vi "ADIS16470 Loop.vi"(8 "error in":errorcluster) -> ()   [LabVIEW 2018]
uses:
  Typedef/ADIS16470 Device Reference.ctl
  Typedef/ADIS16470 Hardware Configuration.ctl
  <vilib>/Rock Robotics/WPI/SPI/WPI_SPIMode.ctl
  <vilib>/Rock Robotics/SystemInterfaces/DIO/FPGA_DIOChannel.ctl
  <vilib>/Rock Robotics/SystemInterfaces/spilib/spi_bus.ctl
  Typedef/ADIS16470 Data.ctl
  Typedef/ADIS16470 Status.ctl
  Typedef/ADIS16470 Process.ctl
  Typedef/ADIS16470 Command Type.ctl
  <vilib>/Rock Robotics/WPI/SPI/WPI_SPIDevRef.ctl
  <vilib>/Rock Robotics/WPI/Interrupt/WPI_InterruptRef.ctl
  <vilib>/Rock Robotics/SystemInterfaces/Interrupt/FPGA_InterruptIndex.ctl
  Typedef/ADIS16470 Register.ctl
  <vilib>/Rock Robotics/WPI/Counter/WPI_CounterDigitalInputToDigitalSource.vi
  <vilib>/Rock Robotics/SystemInterfaces/CounterEncoderSourceConvertion/FPGA_CounterEncoderSourceConvertionLVSourceTypeToFPGAType.vi
  <vilib>/Rock Robotics/WPI/Interrupt/WPI_InterruptCache.vi
  <vilib>/Rock Robotics/SystemInterfaces/Interrupt/FPGA_InterruptWriteConfiguration.vi
  <vilib>/Rock Robotics/SystemInterfaces/Interrupt/FPGA_WaitOnInterrupt.vi
  <vilib>/Rock Robotics/WPI/Utilities/WPI_UtilitiesTimebaseConstants.vi
  <vilib>/Rock Robotics/SystemInterfaces/Interrupt/FPGA_InterruptReadTimestamp.vi
panel:
  out "Waveform Chart":dbl(graph)
  out "Offset Bias":i16[](array[numeric])
  out "xAngle":dbl
  out "yAngle":dbl
  out "Data":dbl[](array[numeric])
  out "Counter":u16
  in  "ADIS16470DevRef":T1={"DevStatus"={"status"=FALSE, "code"=0, "source"=""}, "Hardware Config"={"SPI Clock Rate (Hz)"=1000000.0, "IMU SPI Mode (3)"=enum."Mode 3 (Clk Idle High,Sample on Trailing)", "IMU Reset Pin"=enum."SPI Port CS2", "IMU SPI Bus"=enum."SPI On-Board, CS0", "IMU Data Ready Pin"=enum."SPI Port CS1"}, "End Calibration"=refnum, "Calibration Complete"=refnum, "Data FIFO"=refnum, "Status FIFO"=refnum, "Last Value Reference"=refnum, "Sychronous Process VI"=refnum, "Cmd FIFO"=refnum}
  in  "Main Name":string
  # "x"
  # "y"
  # "z"
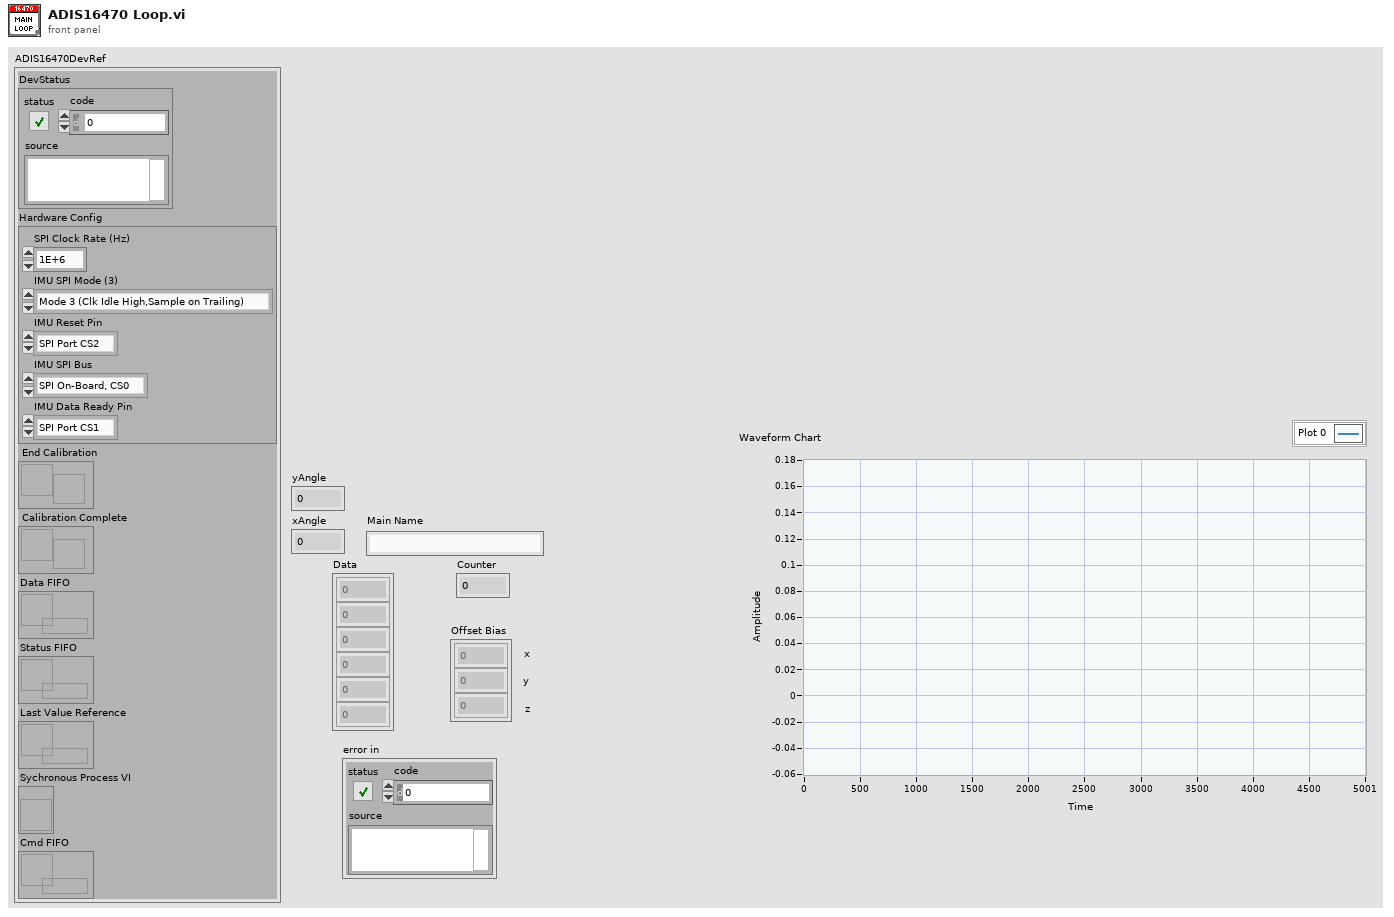
[diagram p1: front panel]
types:
  T1 = typedef "ADIS16470 Device Reference.ctl" = cluster{"DevStatus":errorcluster, "Hardware Config":T2, "End Calibration":refnum<notifier>, "Calibration Complete":refnum<notifier>, "Data FIFO":refnum<k33>, "Status FIFO":refnum<k33>, "Last Value Reference":refnum<data-value>, "Sychronous Process VI":T6, "Cmd FIFO":refnum<k33>}
  T2 = typedef "ADIS16470 Hardware Configuration.ctl" = cluster{"SPI Clock Rate (Hz)":dbl, "IMU SPI Mode (3)":T3, "IMU Reset Pin":T4, "IMU SPI Bus":T5, "IMU Data Ready Pin":T4}
  T3 = typedef "WPI_SPIMode.ctl" = enum16{"Mode 0 (Clk Idle Low,Sample on Leading)", "Mode 1 (Clk Idle Low,Sample on Trailing)", "Mode 2 (Clk Idle High,Sample on Leading)", "Mode 3 (Clk Idle High,Sample on Trailing)"}
  T4 = typedef "FPGA_DIOChannel.ctl" = enum8{"DIO 0", "DIO 1", "DIO 2", "DIO 3", "DIO 4", "DIO 5", "DIO 6", "DIO 7", "DIO 8", "DIO 9", "DIO MXP 0", "DIO MXP 1", "DIO MXP 2", "DIO MXP 3", "DIO MXP 4", "DIO MXP 5", "DIO MXP 6", "DIO MXP 7", "DIO MXP 8", "DIO MXP 9", "DIO MXP 10", "DIO MXP 11", "DIO MXP 12", "DIO MXP 13", "DIO MXP 14", "DIO MXP 15", "SPI Port CS1", "SPI Port CS2", "SPI Port CS3", "SPI Port MISO", "SPI Port MOSI", "Invalid"}
  T5 = typedef "spi_bus.ctl" = enum16{"SPI On-Board, CS0", "SPI On-Board, CS1", "SPI On-Board, CS2", "SPI On-Board, CS3", "SPI MXP", "Invalid"}
  T6 = typedef "ADIS16470 Process.ctl" = refnum<vi>
  T7 = typedef "WPI_SPIDevRef.ctl" = cluster{"DevStatus":errorcluster, "Handle":i32, "SPI Bus":T5}
  T8 = typedef "WPI_InterruptRef.ctl" = cluster{"DevStatus":errorcluster, "InterruptIndex":T9}
  T9 = typedef "FPGA_InterruptIndex.ctl" = enum8{"0", "1", "2", "3", "4", "5", "6", "7", "Invalid"}
  T10 = cluster{"ADIS16470DevRef":T1, "SPIDevRef":T7, "InterruptRef":T8, "Sensor to Robot Rotation":dbl[][], "Yaw":dbl, "Data Counter":u16, "First Run":bool, "TimeStamp Prev":dbl, "Time Delta":dbl}
  T11 = typedef "ADIS16470 Status.ctl" = cluster{"Calibrated?":bool}
  T12 = typedef "ADIS16470 Register.ctl" = u8
  T13 = typedef "ADIS16470 Command Type.ctl" = enum16{"None", "Reset"}
  T14 = typedef "ADIS16470 Data.ctl" = cluster{"Yaw":dbl, "Timestamp":dbl, "Timestamp Delta":dbl, "Sample Count":u16}
  T15 = typedef "WPI_DigitalOutputDevRef.ctl" = cluster{"DIO Channel":T4, "DevStatus":errorcluster}
  T16 = typedef "WPI_DigitalInputDevRef.ctl" = cluster{"DevStatus":errorcluster, "DIO Channel":T4}
  T17 = typedef "FPGA_CounterEncoderSourceConvertionLVSourceType.ctl" = cluster{"DevStatus":errorcluster, "AnalogTriggerMode?":bool, "DigitalMode":cluster{"DIO Channel":T18}, "AnalogTriggerMode":cluster{"AnalogTriggerIndex":T19, "OutputType":T20}}
  T18 = typedef "FPGA_DIODigitalSourceChannel.ctl" = enum8{"DIO 0", "DIO 1", "DIO 2", "DIO 3", "DIO 4", "DIO 5", "DIO 6", "DIO 7", "DIO 8", "DIO 9", "DIO MXP 0", "DIO MXP 1", "DIO MXP 2", "DIO MXP 3", "DIO MXP 4", "DIO MXP 5", "DIO MXP 6", "DIO MXP 7", "DIO MXP 8", "DIO MXP 9", "DIO MXP 10", "DIO MXP 11", "DIO MXP 12", "DIO MXP 13", "DIO MXP 14", "DIO MXP 15", "SPI Port CS1", "SPI Port CS2", "SPI Port CS3", "SPI Port MISO", "SPI Port MOSI", "Disabled"}
  T19 = typedef "FPGA_AnalogTriggerIndex.ctl" = enum8{"Trig 0", "Trig 1", "Trig 2", "Trig 3", "Trig 4", "Trig 5", "Trig 6", "Trig 7", "Invalid"}
  T20 = typedef "FPGA_AnalogTriggerOutType.ctl" = enum16{"InWindow", "TriggerState", "Rising", "Falling"}
  T21 = enum32{"Bad", "Idle", "Run top level", "Running"}
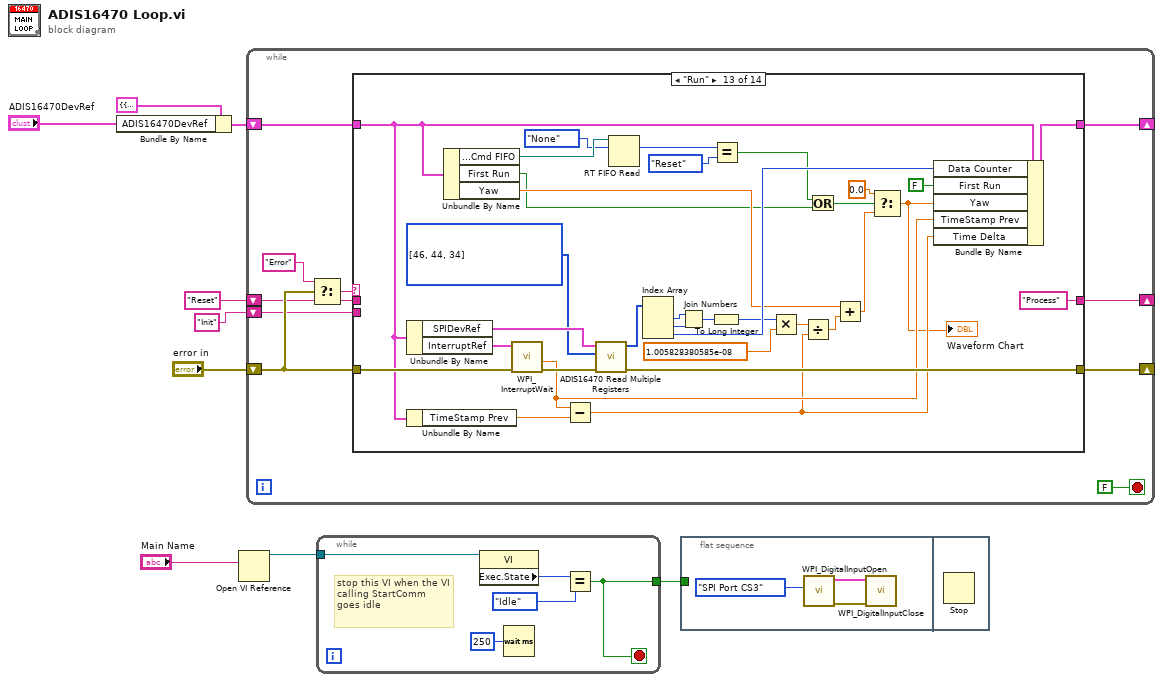
[diagram p0: block diagram]
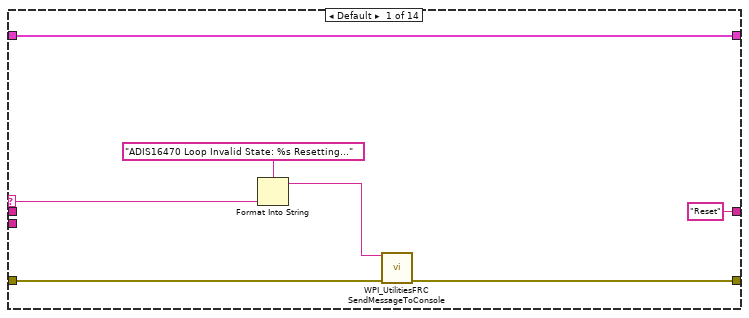
[diagram p2: hidden frame]
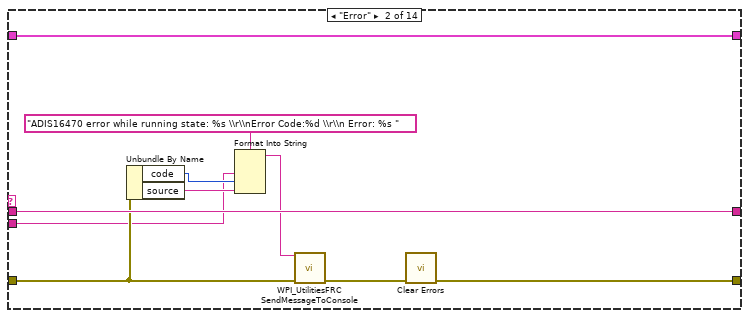
[diagram p3: hidden frame]
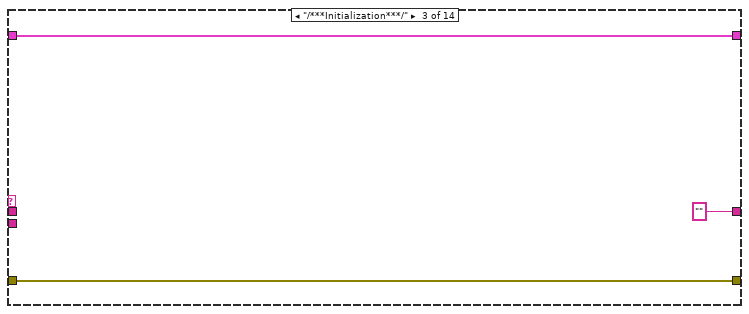
[diagram p4: hidden frame]
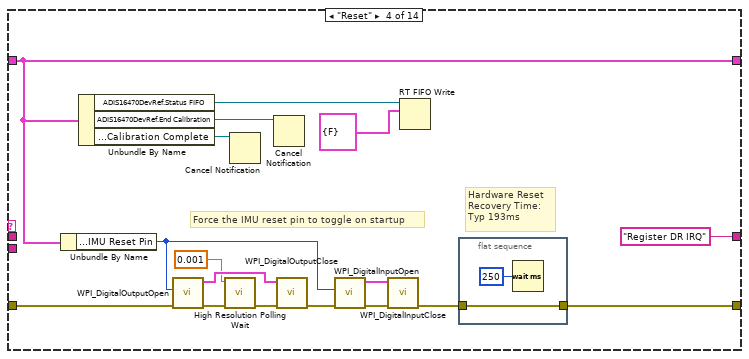
[diagram p5: hidden frame]
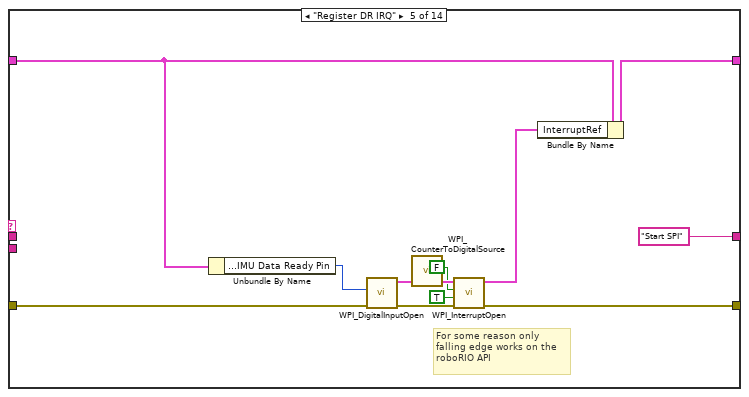
[diagram p6: hidden frame]
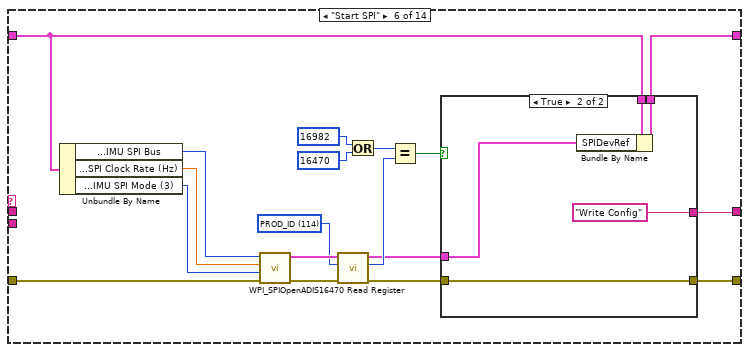
[diagram p7: hidden frame]
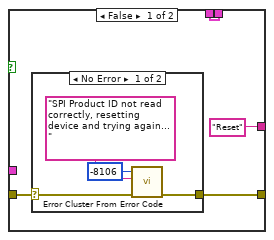
[diagram p8: hidden frame]
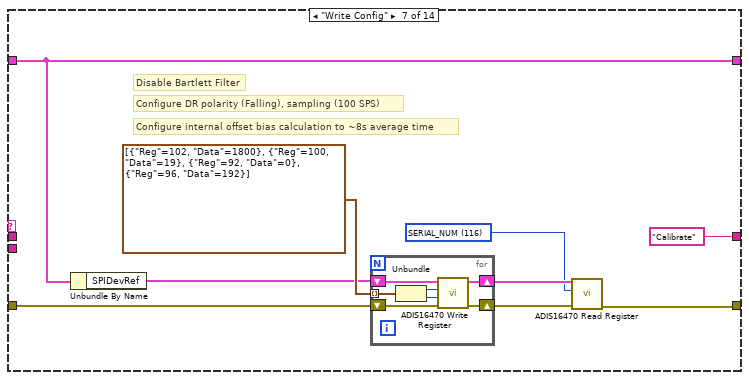
[diagram p10: hidden frame]
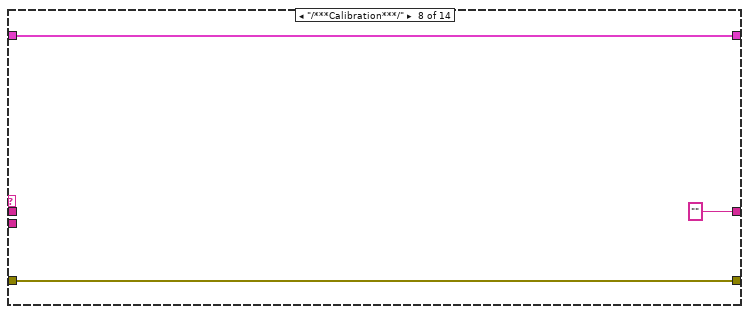
[diagram p11: hidden frame]
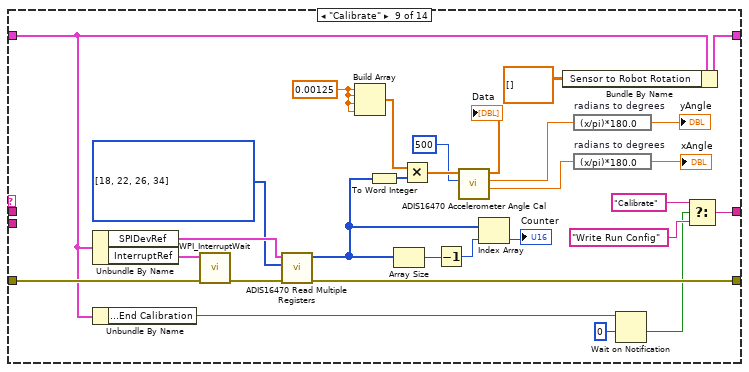
[diagram p12: hidden frame]
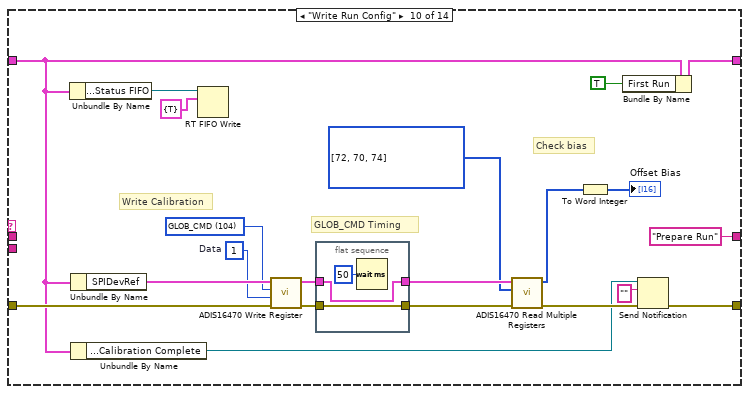
[diagram p13: hidden frame]
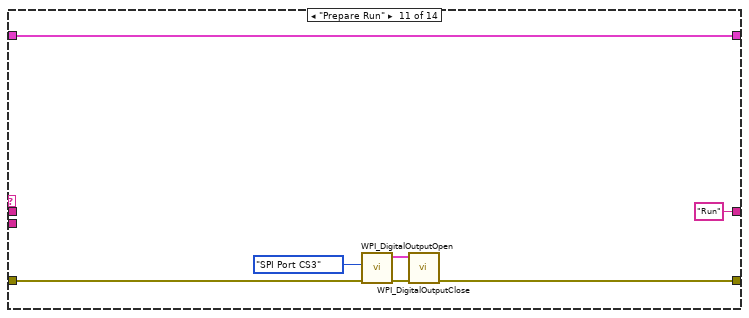
[diagram p14: hidden frame]
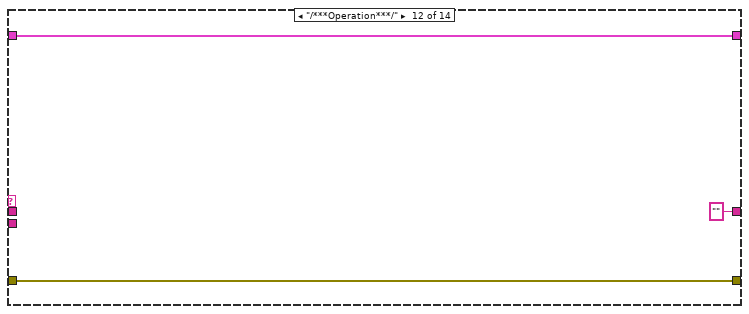
[diagram p15: hidden frame]
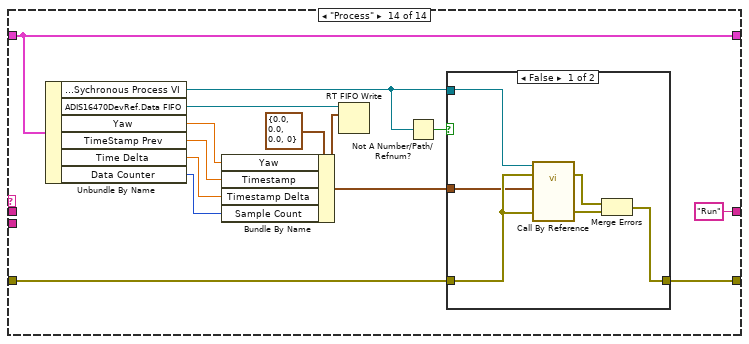
[diagram p16: hidden frame]
diagram:
  n1 = Bundle By Name(cluster=T10 {"ADIS16470DevRef"={"DevStatus"={"status"=FALSE, "code"=0, "source"=""}, "Hardware Config"={"SPI Clock Rate (Hz)"=1000000.0, "IMU SPI Mode (3)"=enum."Mode 3 (Clk Idle High,Sample on Trailing)", "IMU Reset Pin"=enum."SPI Port CS2", "IMU SPI Bus"=enum."SPI On-Board, CS0", "IMU Data Ready Pin"=enum."SPI Port CS1"}, "End Calibration"=refnum, "Calibration Complete"=refnum, "Data FIFO"=refnum, "Status FIFO"=refnum, "Last Value Reference"=refnum, "Sychronous Process VI"=refnum, "Cmd FIFO"=refnum}, "SPIDevRef"={"DevStatus"={"status"=FALSE, "code"=0, "source"=""}, "Handle"=0, "SPI Bus"=enum."SPI On-Board, CS0"}, "InterruptRef"={"DevStatus"={"status"=FALSE, "code"=0, "source"=""}, "InterruptIndex"=enum."Invalid"}, "Sensor to Robot Rotation"=[[0.0, 0.0, 0.0], [0.0, 0.0, 0.0], [0.0, 0.0, 0.0]], "Yaw"=0.0, "Data Counter"=0, "First Run"=FALSE, "TimeStamp Prev"=0.0, "Time Delta"=0.0}, "ADIS16470DevRef"="ADIS16470DevRef") -> (w4:T10)
  n2 = Open VI Reference(vi path="Main Name") -> (vi reference=w8:refnum<vi>)  [unwired: 3 in, 3 out]
  n3 = while {
    shift-right: [w15] -> _
    shift-left: "Reset" -> [w12]
    shift-right: [w17] -> _
    shift-left: w4 -> [w18]
    shift-right: [w16] -> _
    shift-left: "error in" -> [w14]
    shift-left: "Init" -> [w10]
    stop <- FALSE stop-if-true
    n4 = Select(t="Error", s=w14, f=w12) -> (s? t:f=w13:string)
    n5 = case shown="\"Run\"" w13 {
      selector: w13 -> [w25 _ _ _ _ _ _ _ _ _ _ _ _ _]
      tunnel: w18 -> [w26 w36 w39 w44 w62 w78 w110 w121 w134 w154 w181 w184 w203 w229]
      tunnel: [w26 w36 w39 w44 w69 w79 w110 w121 w136 w162 w181 w184 w206 w229] -> w17
      tunnel: w14 -> [w24 w32 w38 w51 w65 w85 w107 w120 w149 w169 w177 w183 w215 w224]
      tunnel: [w23 w33 w38 w46 w68 w77 w104 w120 w146 w156 w176 w183 w212 w222] -> w16
      tunnel: ["Reset" w35 "" "Register DR IRQ" "Start SPI" w80 "Calibrate" "" w133 "Prepare Run" "Run" "" "Process" "Run"] -> w15
      tunnel: w12 -> [_ w35 _ _ _ _ _ _ _ _ _ _ _ _]
      tunnel: w10 -> [_ w27 _ _ _ _ _ _ _ _ _ _ _ _]
      frame Default {
        n6 = Format Into String(format string="ADIS16470 Loop Invalid State: %s Resetting...", w25) -> (resulting string=w22:string)  [unwired: 2 in, 1 out]
        n7 = call <vilib>:"WPI_UtilitiesFRC SendMessageToConsole.vi"("Message"=w22, "error in (no error)"=w24) -> ("error out"=w23:errorcluster)  [unwired: 13 in]
      }
      frame "Error" {
        n8 = Unbundle By Name(w32) -> ("code"=w29:i32, "source"=w28:string)
        n9 = Format Into String(format string="ADIS16470 error while running state: %s \\r\\nError Code:%d \\r\\n Error: %s ", w27, w29, w28) -> (resulting string=w31:string)  [unwired: 2 in, 1 out]
        n10 = call <vilib>:"WPI_UtilitiesFRC SendMessageToConsole.vi"("Message"=w31, "error in (no error)"=w32) -> ("error out"=w34:errorcluster)  [unwired: 13 in]
        n11 = call <vilib>:"Clear Errors.vi"("error in (no error)"=w34) -> ("error out"=w33:errorcluster)  [unwired: 5 in, 1 out]
      }
      frame "/***Initialization***/" {
      }
      frame "Reset" {
        # "Hardware Reset Recovery Time: Typ 193ms"
        # "Force the IMU reset pin to toggle on startup"
        n12 = Unbundle By Name(w44) -> ("ADIS16470DevRef.Hardware Config.IMU Reset Pin"=w52:T4)
        n13 = Unbundle By Name(w44) -> ("ADIS16470DevRef.Status FIFO"=w41:refnum<k33>, "ADIS16470DevRef.End Calibration"=w42:refnum<notifier>, "ADIS16470DevRef.Calibration Complete"=w43:refnum<notifier>)
        n14 = call <vilib>:"WPI_DigitalOutputOpen.vi"("error in (no error)"=w51, "DIO Channel"=w52) -> ("error out"=w49:errorcluster, "DigitalOutputDevRef"=w53:T15)  [unwired: 8 in]
        n15 = call <vilib>:"High Resolution Polling Wait.vi"("error in (no error)"=w49, "seconds to wait"=0.001) -> ("error out"=w48:errorcluster)  [unwired: 9 in]
        n16 = Cancel Notification(0:w43) -> ()  [unwired: 1 in, 3 out]
        n17 = Cancel Notification(0:w42) -> ()  [unwired: 1 in, 3 out]
        n18 = call <vilib>:"WPI_DigitalOutputClose.vi"("error in (no error)"=w48, "DigitalOutputDevRef"=w53) -> ("error out"=w56:errorcluster)  [unwired: 9 in]
        n19 = call <vilib>:"WPI_DigitalInputOpen.vi"("error in (no error)"=w56, "DIO Channel"=w52) -> ("error out"=w55:errorcluster, "DigitalInputDevRef"=w54:T16)  [unwired: 8 in]
        n20 = call <vilib>:"WPI_DigitalInputClose.vi"("error in (no error)"=w55, "DigitalInputDevRef"=w54) -> ("error out"=w45:errorcluster)  [unwired: 9 in]
        n21 = RT FIFO Write(0:w41, 1:T11 {"Calibrated?"=FALSE} ("element")) -> ()  [unwired: 3 in, 4 out]
        n22 = flat-sequence {
          tunnel: [w58] -> w46
          tunnel: w45 -> [w58]
          frame #0 {
            n23 = Wait (ms)(milliseconds to wait=u32 250) -> ()  [unwired: 1 out]
          }
        }
      }
      frame "Register DR IRQ" {
        # "For some reason only\nfalling edge works on the\nroboRIO API"
        n24 = Unbundle By Name(w62) -> ("ADIS16470DevRef.Hardware Config.IMU Data Ready Pin"=w61:T4)
        n25 = call <vilib>:"WPI_DigitalInputOpen.vi"("error in (no error)"=w65, "DIO Channel"=w61) -> ("error out"=w64:errorcluster, "DigitalInputDevRef"=w63:T16)  [unwired: 8 in]
        n26 = call-poly <vilib>:"WPI_CounterToDigitalSource.vi"("DigitalInputDevRef"=w63) -> ("Digital Source"=w66:T17)  [unwired: 6 in]
        n27 = call <vilib>:"WPI_InterruptOpen.vi"("error in (no error)"=w64, "Falling Edge"=TRUE, "Rising Edge"=FALSE, "Source"=w66) -> ("error out"=w68:errorcluster, "InterruptRef"=w67:T8)  [unwired: 6 in]
        n28 = Bundle By Name(cluster=w62, "InterruptRef"=w67) -> (w69:T10)
      }
      frame "Start SPI" {
        w72 = T12 114 items=["Reserved1"=0, "DIAG_STAT"=2, "X_GYRO_LOW"=4, "X_GYRO_OUT"=6, "Y_GYRO_LOW"=8, "Y_GYRO_OUT"=10, "Z_GYRO_LOW"=12, "Z_GYRO_OUT"=14, "X_ACCL_LOW"=16, "X_ACCL_OUT"=18, "Y_ACCL_LOW"=20, "Y_ACCL_OUT"=22, "Z_ACCL_LOW"=24, "Z_ACCL_OUT"=26, "TEMP_OUT"=28, "TIME_STAMP"=30, "Reseved2"=32, "DATA_CNTR"=34, "X_DELTANG_LOW"=36, "X_DELTANG_OUT"=38, "Y_DELTANG_LOW"=40, "Y_DELTANG_OUT"=42, "Z_DELTANG_LOW"=44, "Z_DELTANG_OUT"=46, "X_DELTVEL_LOW"=48, "X_DELTVEL_OUT"=50, "Y_DELTVEL_LOW"=52, "Y_DELTVEL_OUT"=54, "Z_DELTVEL_LOW"=56, "Z_DELTVEL_OUT"=58, "Reserved3"=60, "Reserved4"=62, "XG_BIAS_LOW"=64, "XG_BIAS_HIGH"=66, "YG_BIAS_LOW"=68, "YG_BIAS_OUT"=70, "ZG_BIAS_LOW"=72, "ZG_BIAS_OUT"=74, "XA_BIAS_LOW"=76, "XA_BIAS_HIGH"=78, "YA_BIAS_LOW"=80, "YA_BIAS_OUT"=82, "ZA_BIAS_LOW"=84, "ZA_BIAS_OUT"=86, "Reserved5"=88, "Reserved6"=90, "FILT_CTRL"=92, "Reserved5"=94, "MSC_CTRL"=96, "UP_SCALE"=98, "DEC_RATE"=100, "NULL_CNFG"=102, "GLOB_CMD"=104, "Reserved6"=106, "FIRM_REV"=108, "FIRM_DM"=110, "FIRM_Y"=112, "PROD_ID"=114, "SERIAL_NUM"=116, "USER_SCR1"=118, "USER_SCR2"=120, "USER_SCR3"=122, "FLSHCNT_LOW"=124, "FLSHCNT_HIGH"=126] ("ADIS16448 Register")
        n29 = Unbundle By Name(w78) -> ("ADIS16470DevRef.Hardware Config.IMU SPI Bus"=w81:T5, "ADIS16470DevRef.Hardware Config.SPI Clock Rate (Hz)"=w82:dbl, "ADIS16470DevRef.Hardware Config.IMU SPI Mode (3)"=w83:T3)
        n30 = call <vilib>:"WPI_SPIOpen.vi"("error in"=w85, "Mode (3)"=w83, "Clock Rate (Hz)"=w82, "SPI Bus"=w81) -> ("error out"=w74:errorcluster, "SPIDevRef"=w73:T7)  [unwired: 6 in]
        n31 = call "ADIS16470 Read Register.vi"("error in (no error)"=w74, "ADIS16470 Register"=w72, "SPIDevRef in"=w73) -> ("error out"=w75:errorcluster, "Register Value"=w76:u16, "SPIDevRef out"=w71:T7)  [unwired: 6 in]
        n32 = Or(x=u16 16982 ("y"), y=u16 16470) -> (x .or. y?=w86:u16)
        n33 = Equal?(x=w86, y=w76) -> (x = y?=w84:bool)
        n34 = case shown="True" w84 {
          tunnel: ["Reset" "Write Config"] -> w80
          tunnel: w78 -> [w91 w101]
          tunnel: [w91 w100] -> w79
          tunnel: [w90 w98] -> w77
          tunnel: w75 -> [w89 w98]
          tunnel: w71 -> [_ w99]
          frame False {
            n35 = case shown="No Error" w89 {
              selector: w89 -> [w95 w97]
              tunnel: [w96 w97] -> w90
              frame No Error {
                n36 = call <vilib>:"Error Cluster From Error Code.vi"("error in (no error)"=w95, "error message (\"\")"="SPI Product ID not read correctly, resetting device and trying again..." ("error message (\"\")"), "error code (0)"=-8106) -> ("error out"=w96:errorcluster)  [unwired: 6 in]
              }
              frame Error {
              }
            }
          }
          frame True {
            n37 = Bundle By Name(cluster=w101, "SPIDevRef"=w99) -> (w100:T10)
          }
        }
      }
      frame "Write Config" {
        w103 = T12 116 items=["Reserved1"=0, "DIAG_STAT"=2, "X_GYRO_LOW"=4, "X_GYRO_OUT"=6, "Y_GYRO_LOW"=8, "Y_GYRO_OUT"=10, "Z_GYRO_LOW"=12, "Z_GYRO_OUT"=14, "X_ACCL_LOW"=16, "X_ACCL_OUT"=18, "Y_ACCL_LOW"=20, "Y_ACCL_OUT"=22, "Z_ACCL_LOW"=24, "Z_ACCL_OUT"=26, "TEMP_OUT"=28, "TIME_STAMP"=30, "Reseved2"=32, "DATA_CNTR"=34, "X_DELTANG_LOW"=36, "X_DELTANG_OUT"=38, "Y_DELTANG_LOW"=40, "Y_DELTANG_OUT"=42, "Z_DELTANG_LOW"=44, "Z_DELTANG_OUT"=46, "X_DELTVEL_LOW"=48, "X_DELTVEL_OUT"=50, "Y_DELTVEL_LOW"=52, "Y_DELTVEL_OUT"=54, "Z_DELTVEL_LOW"=56, "Z_DELTVEL_OUT"=58, "Reserved3"=60, "Reserved4"=62, "XG_BIAS_LOW"=64, "XG_BIAS_HIGH"=66, "YG_BIAS_LOW"=68, "YG_BIAS_OUT"=70, "ZG_BIAS_LOW"=72, "ZG_BIAS_OUT"=74, "XA_BIAS_LOW"=76, "XA_BIAS_HIGH"=78, "YA_BIAS_LOW"=80, "YA_BIAS_OUT"=82, "ZA_BIAS_LOW"=84, "ZA_BIAS_OUT"=86, "Reserved5"=88, "Reserved6"=90, "FILT_CTRL"=92, "Reserved5"=94, "MSC_CTRL"=96, "UP_SCALE"=98, "DEC_RATE"=100, "NULL_CNFG"=102, "GLOB_CMD"=104, "Reserved6"=106, "FIRM_REV"=108, "FIRM_DM"=110, "FIRM_Y"=112, "PROD_ID"=114, "SERIAL_NUM"=116, "USER_SCR1"=118, "USER_SCR2"=120, "USER_SCR3"=122, "FLSHCNT_LOW"=124, "FLSHCNT_HIGH"=126] ("ADIS16448 Register")
        # "Configure internal offset bias calculation to ~8s average time"
        # "Configure DR polarity (Falling), sampling (100 SPS)"
        # "Disable Bartlett Filter"
        n38 = Unbundle By Name(w110) -> ("SPIDevRef"=w108:T7)
        n39 = for {
          tunnel: cluster{"Reg":T12, "Data":u16}[] [{"Reg"=102, "Data"=1800}, {"Reg"=100, "Data"=19}, {"Reg"=92, "Data"=0}, {"Reg"=96, "Data"=192}] -> [w118] mode=indexing
          shift-right: [w114] -> w105
          shift-left: w107 -> [w113]
          shift-right: [w112] -> w106
          shift-left: w108 -> [w115]
          n40 = Unbundle(w118) -> ("Reg"=w117:T12, "Data"=w116:u16)
          n41 = call "ADIS16470 Write Register.vi"("error in (no error)"=w113, "Data"=w116, "Register"=w117, "SPIDevRef in"=w115) -> ("error out"=w114:errorcluster, "SPIDevRef out"=w112:T7)  [unwired: 6 in]
        }
        n42 = call "ADIS16470 Read Register.vi"("error in (no error)"=w105, "ADIS16470 Register"=w103, "SPIDevRef in"=w106) -> ("error out"=w104:errorcluster)  [unwired: 6 in, 2 out]
      }
      frame "/***Calibration***/" {
      }
      frame "Calibrate" {
        w140 = 0.00125
        w141 = T12[] [18, 22, 26, 34] items=["Reserved1"=0, "DIAG_STAT"=2, "X_GYRO_LOW"=4, "X_GYRO_OUT"=6, "Y_GYRO_LOW"=8, "Y_GYRO_OUT"=10, "Z_GYRO_LOW"=12, "Z_GYRO_OUT"=14, "X_ACCL_LOW"=16, "X_ACCL_OUT"=18, "Y_ACCL_LOW"=20, "Y_ACCL_OUT"=22, "Z_ACCL_LOW"=24, "Z_ACCL_OUT"=26, "TEMP_OUT"=28, "TIME_STAMP"=30, "Reseved2"=32, "DATA_CNTR"=34, "X_DELTANG_LOW"=36, "X_DELTANG_OUT"=38, "Y_DELTANG_LOW"=40, "Y_DELTANG_OUT"=42, "Z_DELTANG_LOW"=44, "Z_DELTANG_OUT"=46, "X_DELTVEL_LOW"=48, "X_DELTVEL_OUT"=50, "Y_DELTVEL_LOW"=52, "Y_DELTVEL_OUT"=54, "Z_DELTVEL_LOW"=56, "Z_DELTVEL_OUT"=58, "Reserved3"=60, "Reserved4"=62, "XG_BIAS_LOW"=64, "XG_BIAS_HIGH"=66, "YG_BIAS_LOW"=68, "YG_BIAS_OUT"=70, "ZG_BIAS_LOW"=72, "ZG_BIAS_OUT"=74, "XA_BIAS_LOW"=76, "XA_BIAS_HIGH"=78, "YA_BIAS_LOW"=80, "YA_BIAS_OUT"=82, "ZA_BIAS_LOW"=84, "ZA_BIAS_OUT"=86, "Reserved5"=88, "Reserved6"=90, "FILT_CTRL"=92, "Reserved5"=94, "MSC_CTRL"=96, "UP_SCALE"=98, "DEC_RATE"=100] ("Registers")
        n43 = Unbundle By Name(w134) -> ("SPIDevRef"=w147:T7, "InterruptRef"=w150:T8)
        n44 = Unbundle By Name(w134) -> ("ADIS16470DevRef.End Calibration"=w124:refnum<notifier>)
        n45 = call <vilib>:"WPI_InterruptWait.vi"("error in (no error)"=w149, "InterruptRef"=w150) -> ("error out"=w148:errorcluster)  [unwired: 5 in, 4 out]
        n46 = call "ADIS16470 Read Multiple Registers.vi"("error in (no error)"=w148, "Registers"=w141, "SPIDevRef"=w147) -> ("error out"=w146:errorcluster, "Values"=w129:u16[])  [unwired: 7 in]
        n47 = Build Array(w140, w140, w140, w140) -> (w145:dbl[])
        n48 = To Word Integer(number=w129) -> (16bit integer=w130:i16[])
        n49 = Array Size(array=w129) -> (size(s)=w144:i32)
        n50 = Multiply(x=w145, y=w130) -> (x*y=w139:dbl[])
        n51 = Decrement(x=w144) -> (x-1=w143:i32)
        n52 = call "ADIS16470 Accelerometer Angle Cal.vi"("average samples"=500, "Raw Accel In"=w139) -> ("xAngle"=w127:dbl, "yAngle"=w126:dbl, "Average Accel Out"=→"Data":dbl[])  [unwired: 7 in]
        n53 = Index Array(array=w129, index=w143) -> (element=→"Counter":u16)
        n54 = Bundle By Name(cluster=w134, "Sensor to Robot Rotation"=dbl[][] []) -> (w136:T10)
        n55 = expression code="(x/pi)*180.0" "radians to degrees"(w126) -> (→"yAngle":dbl)
        n56 = expression code="(x/pi)*180.0" "radians to degrees"(w127) -> (→"xAngle":dbl)
        n57 = Wait on Notification(notifier=w124, timeout in ms (-1)=0) -> (timed out?=w122:bool)  [unwired: 2 in, 3 out]
        n58 = Select(t="Calibrate", s=w122, f="Write Run Config") -> (s? t:f=w133:string)
      }
      frame "Write Run Config" {
        w151 = T12 104 items=["Reserved1"=0, "DIAG_STAT"=2, "X_GYRO_LOW"=4, "X_GYRO_OUT"=6, "Y_GYRO_LOW"=8, "Y_GYRO_OUT"=10, "Z_GYRO_LOW"=12, "Z_GYRO_OUT"=14, "X_ACCL_LOW"=16, "X_ACCL_OUT"=18, "Y_ACCL_LOW"=20, "Y_ACCL_OUT"=22, "Z_ACCL_LOW"=24, "Z_ACCL_OUT"=26, "TEMP_OUT"=28, "TIME_STAMP"=30, "Reseved2"=32, "DATA_CNTR"=34, "X_DELTANG_LOW"=36, "X_DELTANG_OUT"=38, "Y_DELTANG_LOW"=40, "Y_DELTANG_OUT"=42, "Z_DELTANG_LOW"=44, "Z_DELTANG_OUT"=46, "X_DELTVEL_LOW"=48, "X_DELTVEL_OUT"=50, "Y_DELTVEL_LOW"=52, "Y_DELTVEL_OUT"=54, "Z_DELTVEL_LOW"=56, "Z_DELTVEL_OUT"=58, "Reserved3"=60, "Reserved4"=62, "XG_BIAS_LOW"=64, "XG_BIAS_HIGH"=66, "YG_BIAS_LOW"=68, "YG_BIAS_OUT"=70, "ZG_BIAS_LOW"=72, "ZG_BIAS_OUT"=74, "XA_BIAS_LOW"=76, "XA_BIAS_HIGH"=78, "YA_BIAS_LOW"=80, "YA_BIAS_OUT"=82, "ZA_BIAS_LOW"=84, "ZA_BIAS_OUT"=86, "Reserved5"=88, "Reserved6"=90, "FILT_CTRL"=92, "Reserved5"=94, "MSC_CTRL"=96, "UP_SCALE"=98, "DEC_RATE"=100, "NULL_CNFG"=102, "GLOB_CMD"=104, "Reserved6"=106, "FIRM_REV"=108, "FIRM_DM"=110, "FIRM_Y"=112, "PROD_ID"=114, "SERIAL_NUM"=116, "USER_SCR1"=118, "USER_SCR2"=120, "USER_SCR3"=122, "FLSHCNT_LOW"=124, "FLSHCNT_HIGH"=126] ("Register")
        w168 = u16 1  # Data
        w163 = T12[] [72, 70, 74] items=["Reserved1"=0, "DIAG_STAT"=2, "X_GYRO_LOW"=4, "X_GYRO_OUT"=6, "Y_GYRO_LOW"=8, "Y_GYRO_OUT"=10, "Z_GYRO_LOW"=12, "Z_GYRO_OUT"=14, "X_ACCL_LOW"=16, "X_ACCL_OUT"=18, "Y_ACCL_LOW"=20, "Y_ACCL_OUT"=22, "Z_ACCL_LOW"=24, "Z_ACCL_OUT"=26, "TEMP_OUT"=28, "TIME_STAMP"=30, "Reseved2"=32, "DATA_CNTR"=34, "X_DELTANG_LOW"=36, "X_DELTANG_OUT"=38, "Y_DELTANG_LOW"=40, "Y_DELTANG_OUT"=42, "Z_DELTANG_LOW"=44, "Z_DELTANG_OUT"=46, "X_DELTVEL_LOW"=48, "X_DELTVEL_OUT"=50, "Y_DELTVEL_LOW"=52, "Y_DELTVEL_OUT"=54, "Z_DELTVEL_LOW"=56, "Z_DELTVEL_OUT"=58, "Reserved3"=60, "Reserved4"=62, "XG_BIAS_LOW"=64, "XG_BIAS_HIGH"=66, "YG_BIAS_LOW"=68, "YG_BIAS_OUT"=70, "ZG_BIAS_LOW"=72, "ZG_BIAS_OUT"=74, "XA_BIAS_LOW"=76, "XA_BIAS_HIGH"=78, "YA_BIAS_LOW"=80, "YA_BIAS_OUT"=82, "ZA_BIAS_LOW"=84, "ZA_BIAS_OUT"=86, "Reserved5"=88, "Reserved6"=90, "FILT_CTRL"=92, "Reserved5"=94, "MSC_CTRL"=96, "UP_SCALE"=98, "DEC_RATE"=100] ("Registers")
        # "Write Calibration"
        # "GLOB_CMD Timing"
        # "Check bias"
        n59 = Unbundle By Name(w154) -> ("ADIS16470DevRef.Status FIFO"=w153:refnum<k33>)
        n60 = Unbundle By Name(w154) -> ("SPIDevRef"=w170:T7)
        n61 = Unbundle By Name(w154) -> ("ADIS16470DevRef.Calibration Complete"=w157:refnum<notifier>)
        n62 = RT FIFO Write(0:w153, 1:T11 {"Calibrated?"=TRUE} ("element")) -> ()  [unwired: 3 in, 4 out]
        n63 = call "ADIS16470 Write Register.vi"("error in (no error)"=w169, "Data"=w168, "Register"=w151, "SPIDevRef in"=w170) -> ("error out"=w167:errorcluster, "SPIDevRef out"=w166:T7)  [unwired: 6 in]
        n64 = flat-sequence {
          tunnel: w167 -> [w174]
          tunnel: [w174] -> w165
          tunnel: w166 -> [w172]
          tunnel: [w172] -> w164
          frame #0 {
            n65 = Wait (ms)(milliseconds to wait=u32 50) -> ()  [unwired: 1 out]
          }
        }
        n66 = call "ADIS16470 Read Multiple Registers.vi"("error in (no error)"=w165, "Registers"=w163, "SPIDevRef"=w164) -> ("error out"=w158:errorcluster, "Values"=w160:u16[])  [unwired: 7 in]
        n67 = To Word Integer(number=w160) -> (16bit integer=→"Offset Bias":i16[])
        n68 = Bundle By Name(cluster=w154, "First Run"=TRUE) -> (w162:T10)
        n69 = Send Notification(notification="", notifier=w157, error in (no error)=w158) -> (error out=w156:errorcluster)  [unwired: 1 out]
      }
      frame "Prepare Run" {
        n70 = call <vilib>:"WPI_DigitalOutputOpen.vi"("error in (no error)"=w177, "DIO Channel"=FPGA_DIOChannel."SPI Port CS3") -> ("error out"=w179:errorcluster, "DigitalOutputDevRef"=w180:T15)  [unwired: 8 in]
        n71 = call <vilib>:"WPI_DigitalOutputClose.vi"("error in (no error)"=w179, "DigitalOutputDevRef"=w180) -> ("error out"=w176:errorcluster)  [unwired: 9 in]
      }
      frame "/***Operation***/" {
      }
      frame "Run" {
        w211 = T12[] [46, 44, 34] items=["Reserved1"=0, "DIAG_STAT"=2, "X_GYRO_LOW"=4, "X_GYRO_OUT"=6, "Y_GYRO_LOW"=8, "Y_GYRO_OUT"=10, "Z_GYRO_LOW"=12, "Z_GYRO_OUT"=14, "X_ACCL_LOW"=16, "X_ACCL_OUT"=18, "Y_ACCL_LOW"=20, "Y_ACCL_OUT"=22, "Z_ACCL_LOW"=24, "Z_ACCL_OUT"=26, "TEMP_OUT"=28, "TIME_STAMP"=30, "Reseved2"=32, "DATA_CNTR"=34, "X_DELTANG_LOW"=36, "X_DELTANG_OUT"=38, "Y_DELTANG_LOW"=40, "Y_DELTANG_OUT"=42, "Z_DELTANG_LOW"=44, "Z_DELTANG_OUT"=46, "X_DELTVEL_LOW"=48, "X_DELTVEL_OUT"=50, "Y_DELTVEL_LOW"=52, "Y_DELTVEL_OUT"=54, "Z_DELTVEL_LOW"=56, "Z_DELTVEL_OUT"=58, "Reserved3"=60, "Reserved4"=62, "XG_BIAS_LOW"=64, "XG_BIAS_HIGH"=66, "YG_BIAS_LOW"=68, "YG_BIAS_OUT"=70, "ZG_BIAS_LOW"=72, "ZG_BIAS_OUT"=74, "XA_BIAS_LOW"=76, "XA_BIAS_HIGH"=78, "YA_BIAS_LOW"=80, "YA_BIAS_OUT"=82, "ZA_BIAS_LOW"=84, "ZA_BIAS_OUT"=86, "Reserved5"=88, "Reserved6"=90, "FILT_CTRL"=92, "Reserved5"=94, "MSC_CTRL"=96, "UP_SCALE"=98, "DEC_RATE"=100] ("Registers")
        n72 = Unbundle By Name(w203) -> ("SPIDevRef"=w214:T7, "InterruptRef"=w216:T8)
        n73 = Unbundle By Name(w203) -> ("TimeStamp Prev"=w197:dbl)
        n74 = Unbundle By Name(w203) -> ("ADIS16470DevRef.Cmd FIFO"=w191:refnum<k33>, "First Run"=w185:bool, "Yaw"=w200:dbl)
        n75 = call <vilib>:"WPI_InterruptWait.vi"("error in (no error)"=w215, "InterruptRef"=w216) -> ("error out"=w213:errorcluster, "TimeStamp"=w196:dbl)  [unwired: 5 in, 3 out]
        n76 = Subtract(x=w196, y=w197) -> (x-y=w193:dbl)
        n77 = call "ADIS16470 Read Multiple Registers.vi"("error in (no error)"=w213, "Registers"=w211, "SPIDevRef"=w214) -> ("error out"=w212:errorcluster, "Values"=w210:u16[])  [unwired: 7 in]
        n78 = RT FIFO Read(0:w191, 1:ADIS16470_Command_Type."None" ("element")) -> (9:w189:T13)  [unwired: 2 in, 4 out]
        n79 = Index Array(array=w210) -> (element #1=w209:u16, element #2=w208:u16, element #3=w205:u16)  [unwired: 3 in]
        n80 = Join Numbers(hi=w209, lo=w208) -> ((hi.lo)=w195:u32)
        n81 = To Long Integer(number=w195) -> (32bit integer=w194:i32)
        n82 = Equal?(x=w189, y=ADIS16470_Command_Type."Reset" ("element")) -> (x = y?=w186:bool)
        n83 = Multiply(x=w194, y=1.005828380585e-08) -> (x*y=w202:dbl)
        n84 = Divide(x=w202, y=w193) -> (x/y=w201:dbl)
        n85 = Or(x=w186, y=w185) -> (x .or. y?=w187:bool)
        n86 = Add(x=w200, y=w201) -> (x+y=w198:dbl)
        n87 = Select(t=0.0, s=w187, f=w198) -> (s? t:f=w192:dbl)
        "Waveform Chart" <- w192
        n88 = Bundle By Name(cluster=w203, "Data Counter"=w205, "First Run"=FALSE, "Yaw"=w192, "TimeStamp Prev"=w196, "Time Delta"=w193) -> (w206:T10)
      }
      frame "Process" {
        n89 = Unbundle By Name(w229) -> ("ADIS16470DevRef.Sychronous Process VI"=w220:T6, "ADIS16470DevRef.Data FIFO"=w228:refnum<k33>, "Yaw"=w225:dbl, "TimeStamp Prev"=w226:dbl, "Time Delta"=w218:dbl, "Data Counter"=w219:u16)
        n90 = Bundle By Name(cluster=T14 {"Yaw"=0.0, "Timestamp"=0.0, "Timestamp Delta"=0.0, "Sample Count"=0} ("element"), "Yaw"=w225, "Timestamp"=w226, "Timestamp Delta"=w218, "Sample Count"=w219) -> (w223:T14)
        n91 = RT FIFO Write(0:w228, 1:w223) -> ()  [unwired: 3 in, 4 out]
        n92 = Not A Number/Path/Refnum?(number/path/refnum=w220) -> (NaN/Path/Refnum?=w221:bool)
        n93 = case shown="False" w221 {
          tunnel: w224 -> [w236 w237]
          tunnel: w223 -> [w235 _]
          tunnel: [w232 w237] -> w222
          tunnel: w220 -> [w231 _]
          frame False {
            n94 = call-by-ref "?"(reference=w231, error in=w236, 8:"error in (no error)"=w236, "element"=w235) -> (error out=w234:errorcluster, 0:"error out"=w233:errorcluster)  [unwired: 9 in, 1 out]
            n95 = Merge Errors(w234, w233) -> (w232:errorcluster)
          }
          frame True {
          }
        }
      }
    }
  }
  n96 = while {
    tunnel: w8 -> [w239]
    tunnel: [w238] -> w1
    stop <- w238 stop-if-true
    # "stop this VI when the VI calling StartComm goes idle"
    n97 = property class="VI"(reference=w239) -> ("Exec.State"=w241:T21)  [unwired: 1 in, 2 out]
    n98 = Wait (ms)(milliseconds to wait=u32 250) -> ()  [unwired: 1 out]
    n99 = Equal?(x=w241, y=T21."Idle" ("Execution:State")) -> (x = y?=w238:bool)
  }
  n100 = flat-sequence {
    tunnel: w1 -> [_]
    frame #0 {
      n101 = call <vilib>:"WPI_DigitalInputOpen.vi"("DIO Channel"=FPGA_DIOChannel."SPI Port CS3") -> ("error out"=w243:errorcluster, "DigitalInputDevRef"=w244:T16)  [unwired: 9 in]
      n102 = call <vilib>:"WPI_DigitalInputClose.vi"("error in (no error)"=w243, "DigitalInputDevRef"=w244) -> ()  [unwired: 9 in, 1 out]
    }
    frame #1 {
      n103 = Stop() -> ()  [unwired: 1 in]
    }
  }
